vi "Configure IQ Recorder Measurement Trigger Timeout State.vi"(8 "error in (no error)":errorcluster, 9 "State (Off)":bool, 10 "Instance (1)":i32=1, 11 "VISA resource name":refnum<visa-resource-name>) -> (0 "error out":errorcluster, 3 "VISA resource name out":refnum<visa-resource-name>)   [LabVIEW 2015, in "Rohde&Schwarz CMXP GPRF.lvlib"]
doc: "Disables timeout | enables timeout using the previous/default values.\n\nAttribute:\nRSCMXPGPRF_ATTR_IQ_RECORDER_MEASUREMENT_TRIGGER_TIMEOUT_ENABLED\n\nRemote-control command:\nTRIGger:GPRF:MEAS<i>:IQRecorder:TOUT"
uses:
  <instrlib>/Rohde&Schwarz CMXP GPRF/Rohde&Schwarz CMXP GPRF.lvlib
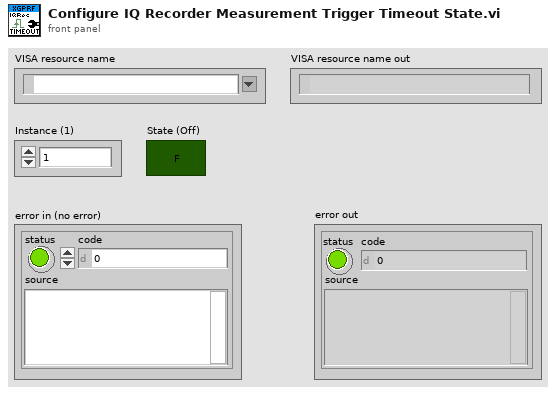
[diagram p1: front panel]
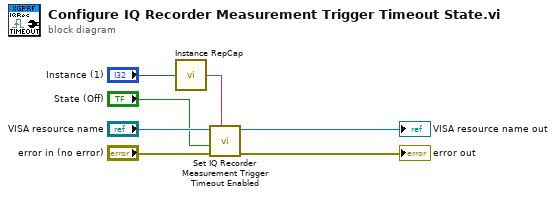
[diagram p0: block diagram]
diagram:
  n1 = call <instrlib>:"Instance RepCap.vi"("instance  in"="Instance (1)") -> ("instance out"=w7:string)
  n2 = call "Set IQ Recorder Measurement Trigger Timeout Enabled"("Repeated Capabilities"=w7, "error in (no error)"="error in (no error)", "IQ Recorder Measurement Trigger Timeout Enabled (OFF)"="State (Off)", "instrument handle"="VISA resource name") -> ("error out"=→"error out":errorcluster, "instrument handle out"=→"VISA resource name out":refnum<visa-resource-name>)  [unwired: 6 in]
